vi "Get LabVIEW Directory.vi"(8 "error in":errorcluster) -> (0 "error out":errorcluster, 3 "LabVIEW Directory":string)   [LabVIEW 2019, in "SEECD System Explorer.lvlib"]
uses:
  SEECD System Explorer.lvlib
  <vilib>/registry/registry.llb/Registry RtKey.ctl
  <vilib>/registry/registry.llb/Registry SAM.ctl
  <vilib>/registry/registry.llb/Read Registry Value Simple STR.vi
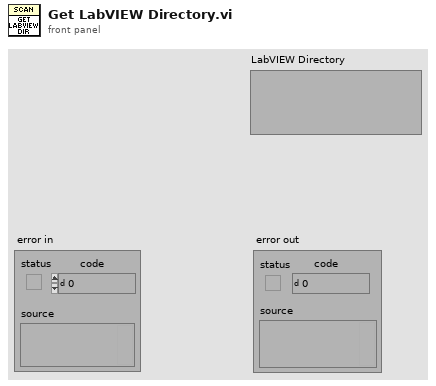
[diagram p1: front panel]
types:
  T1 = typedef "Registry SAM.ctl" = enum32{"KEY_QUERY_VALUE", "KEY_SET_VALUE", "KEY_CREATE_SUB_KEY", "KEY_ENUMERATE_SUB_KEYS", "KEY_NOTIFY", "KEY_CREATE_LINK", "KEY_READ", "KEY_WRITE", "KEY_ALL_ACCESS", "KEY_READ | KEY_WRITE"}
  T2 = typedef "Registry RtKey.ctl" = enum32{"HKEY_CLASSES_ROOT", "HKEY_CURRENT_USER", "HKEY_LOCAL_MACHINE", "HKEY_USERS", "HKEY_PERFORMANCE_DATA", "HKEY_CURRENT_CONFIG", "HKEY_DYN_DATA"}
  T3 = typedef "Registry refnum.ctl" = refnum<k1>
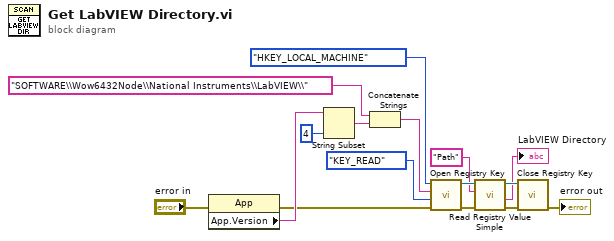
[diagram p0: block diagram]
diagram:
  n1 = property class="App"(error in="error in") -> (error out=w1:errorcluster, "App.Version"=w7:string)  [unwired: 1 in, 1 out]
  n2 = String Subset(string=w7, length (rest)=4 ("length (rest)")) -> (substring=w4:string)  [unwired: 1 in]
  n3 = Concatenate Strings("SOFTWARE\\Wow6432Node\\National Instruments\\LabVIEW\\", w4) -> (w3:string)
  n4 = call <vilib>:"Open Registry Key.vi"("error in (no error)"=w1, "security access mask (KEY_READ | KEY_WRITE)"=Registry_SAM."KEY_READ", "subkey"=w3, "root key (HKEY_LOCAL_MACHINE)"=Registry_RtKey."HKEY_LOCAL_MACHINE") -> ("error out"=w12:errorcluster, "refnum out"=w11:T3)  [unwired: 6 in]
  n5 = call-poly <vilib>:"Read Registry Value Simple.vi"("error in (no error)"=w12, "value"="Path", "refnum"=w11) -> ("error out"=w16:errorcluster, "String/Binary data"=→"LabVIEW Directory":string, "refnum out"=w15:T3)  [unwired: 3 in, 1 out]
  n6 = call <vilib>:"Close Registry Key.vi"("error in (no error)"=w16, "refnum"=w15) -> ("error out"=→"error out":errorcluster)  [unwired: 5 in]
